vi "FPGA - Select Bitfile (ECAT).vi"(8 "error in (no error)":errorcluster, 11 "Node Ptr":u64 format="%.0x") -> (0 "error out":errorcluster)   [LabVIEW 2016, in "Scan Engine Custom Device.lvlib"]
uses:
  Scan Engine Custom Device.lvlib
  Type Defs/FPGA Target.ctl
  <vilib>/NI Veristand/Custom Device Tools/Custom Device Utility Library/Custom Device Utility Library.lvlib
panel:
  in  "Tag":string
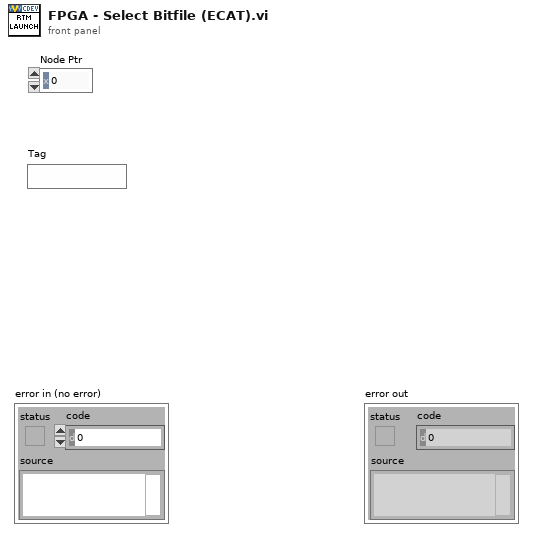
[diagram p1: front panel]
types:
  T1 = typedef "Scan Engine Custom Device.lvlib/FPGA Target.ctl" = enum16{"Local", "EtherCAT"}
  T2 = typedef "Custom Device API.lvlib/Custom Device Item Ref.ctl" = u64
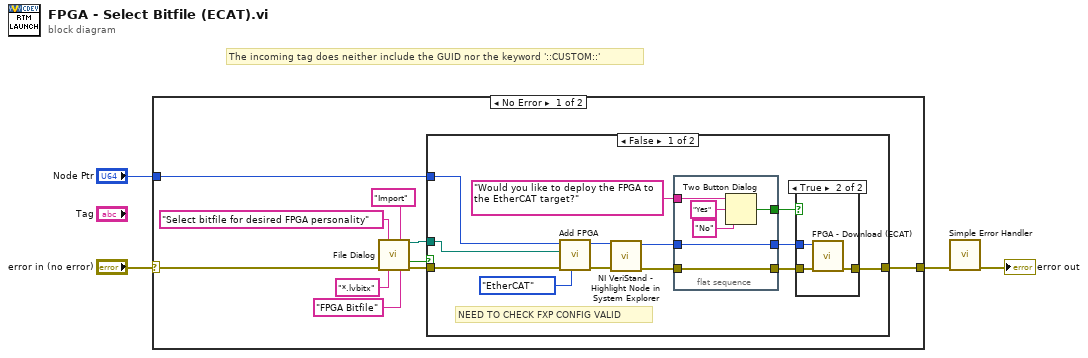
[diagram p0: block diagram]
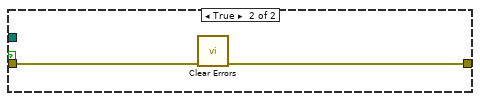
[diagram p3: hidden frame]
diagram:
  # "The incoming tag does neither include the GUID nor the keyword '::CUSTOM::'"
  n1 = case shown="No Error" "error in (no error)" {
    selector: "error in (no error)" -> [w6 w40]
    tunnel: "Node Ptr" -> [w5 _]
    tunnel: [w7 w40] -> w2
    frame No Error {
      n2 = call "File Dialog"("prompt"="Select bitfile for desired FPGA personality", "button label"="Import", "error in"=w6, "pattern (all files)"="*.lvbitx", "pattern label"="FPGA Bitfile") -> ("selected path"=w14:path, "cancelled"=w12:bool, "error out"=w13:errorcluster)  [unwired: 7 in, 1 out]
      n3 = case shown="False" w12 {
        tunnel: w13 -> [w24 w39]
        tunnel: w14 -> [w26 _]
        tunnel: [w15 w38] -> w7
        tunnel: w5 -> [w27 _]
        frame False {
          # "NEED TO CHECK FXP CONFIG VALID"
          n4 = call "Add FPGA.vi"("FPGA Target"=FPGA_Target."EtherCAT", "error in (no error)"=w24, "Bitfile Path"=w26, "Item Ref in"=w27) -> ("error out"=w23:errorcluster, "Item Ref out"=w22:T2)  [unwired: 6 in]
          n5 = call <vilib>:"NI VeriStand - Highlight Node in System Explorer.vi"("error in (no error)"=w23, "Item Ref in"=w22) -> ("error out"=w21:errorcluster, "Node Ptr dup"=w17:T2)  [unwired: 8 in]
          n6 = flat-sequence {
            tunnel: w21 -> [w35]
            tunnel: [w35] -> w19
            tunnel: "Would you like to deploy the FPGA to the EtherCAT target?" ("message") -> [w34]
            tunnel: [w33] -> w18
            tunnel: w17 -> [w33]
            tunnel: [w32] -> w16
            frame #0 {
              n7 = Two Button Dialog(message=w34, 1:"No" ("F button name (\"Cancel\")"), 2:"Yes" ("T button name (\"OK\")")) -> (T button?=w32:bool)
            }
          }
          n8 = case shown="True" w16 {
            tunnel: w19 -> [w28 w31]
            tunnel: w18 -> [_ w30]
            tunnel: [w28 w29] -> w15
            frame False {
            }
            frame True {
              n9 = call "FPGA - Download (ECAT).vi"("error in (no error)"=w31, "Node Ptr"=w30) -> ("error out"=w29:errorcluster)  [unwired: 9 in]
            }
          }
        }
        frame True {
          n10 = call <vilib>:"Clear Errors.vi"("error in (no error)"=w39) -> ("error out"=w38:errorcluster)  [unwired: 1 in, 5 out]
        }
      }
    }
    frame Error {
    }
  }
  n11 = call <vilib>:"Simple Error Handler.vi"("error in (no error)"=w2) -> ("error out"=→"error out":errorcluster)  [unwired: 4 in, 4 out]
